vi "Write Config.vi"(8 "error in (no error)":errorcluster, 10 "Config":variant, 11 "Plugin in":refnum<class "Plugin.lvclass">) -> (0 "error out":errorcluster, 3 "Plugin out":refnum<class "Plugin.lvclass">)   [LabVIEW 2015, in "Plugin.lvclass"]
uses:
  Plugin.lvclass
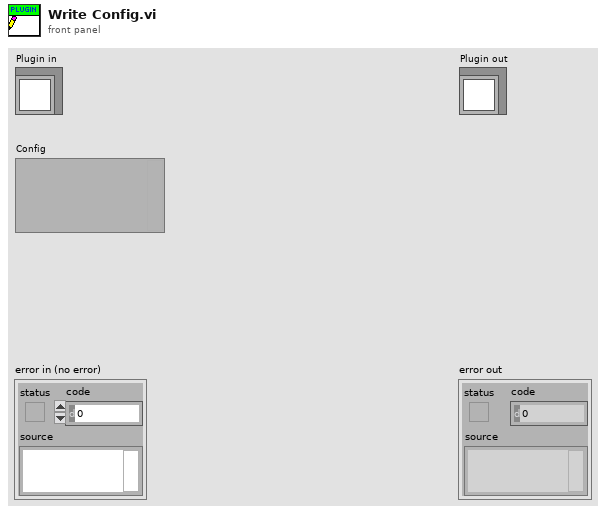
[diagram p1: front panel]
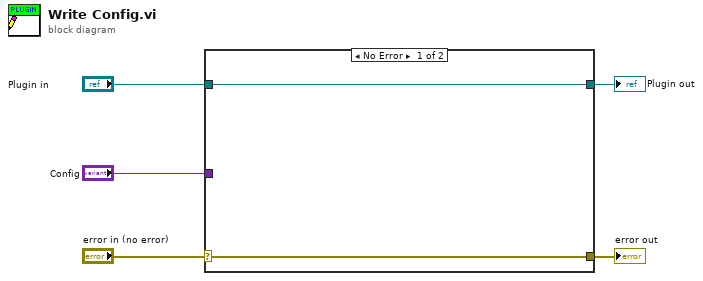
[diagram p0: block diagram]
diagram:
  n1 = case shown="No Error" "error in (no error)" {
    selector: "error in (no error)" -> [w7 w8]
    tunnel: [w7 w8] -> w4
    tunnel: [w6 w9] -> w2
    tunnel: "Plugin in" -> [w6 w9]
    tunnel: "Config" -> [_ _]
    frame No Error {
    }
    frame Error {
    }
  }
  "error out" <- w4
  "Plugin out" <- w2
